vi "Can_File_be_Editted.vi"(0 "Filename":path) -> (1 "File Permissions OK?":bool, 2 "File Status":T1=enum."Directory structure cannot be created", 3 "Comment String":string="Directory structure cannot be created", 4 "Cannot create directory":path)   [LabVIEW 2010]
uses:
  File_Status.ctl
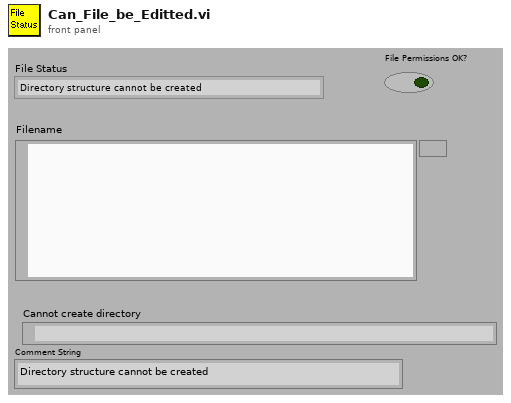
[diagram p1: front panel]
types:
  T1 = typedef "File_Status.ctl" = enum16{"Invalid Path", "This is a folder pathname", "Generic File Error", "Directory structure cannot be created", "File cannot be created", "File can be created", "File exist but read only", "File exist but no access", "File exist with read and write access"}
  T2 = enum16{"read/write", "read-only", "write-only", "write-only (truncate)"}
  T3 = enum16{"open", "replace", "create", "open or create", "replace or create", "replace or create with confirmation"}
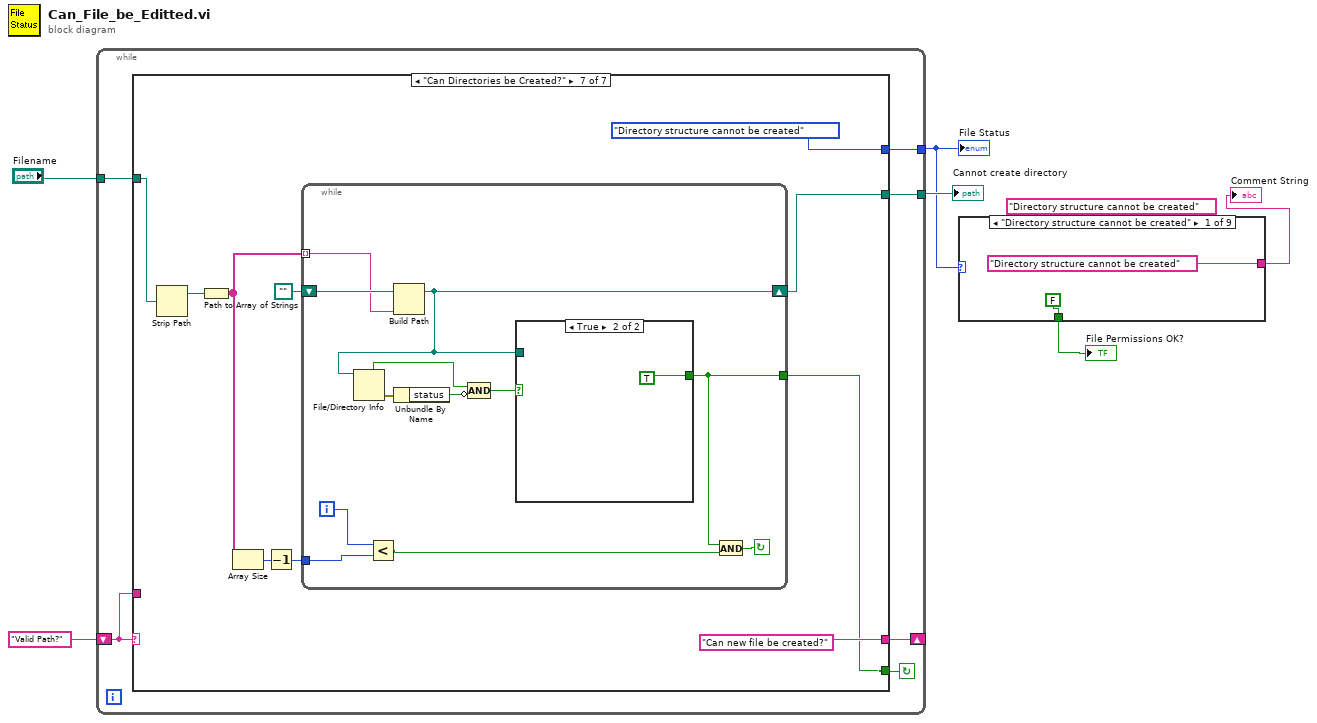
[diagram p0: block diagram]
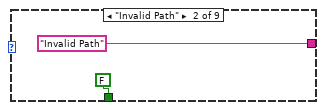
[diagram p2: hidden frame]
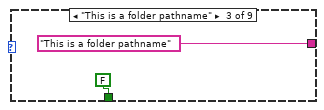
[diagram p3: hidden frame]
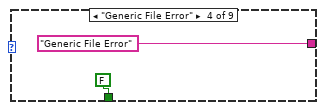
[diagram p4: hidden frame]
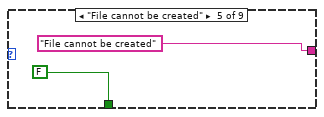
[diagram p5: hidden frame]
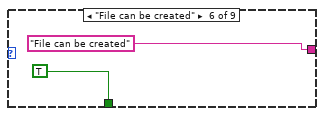
[diagram p6: hidden frame]
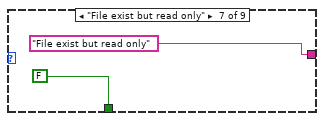
[diagram p7: hidden frame]
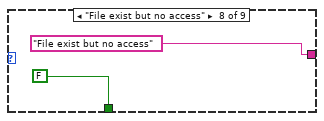
[diagram p8: hidden frame]
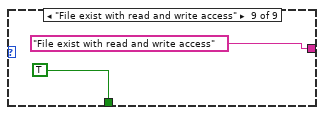
[diagram p9: hidden frame]
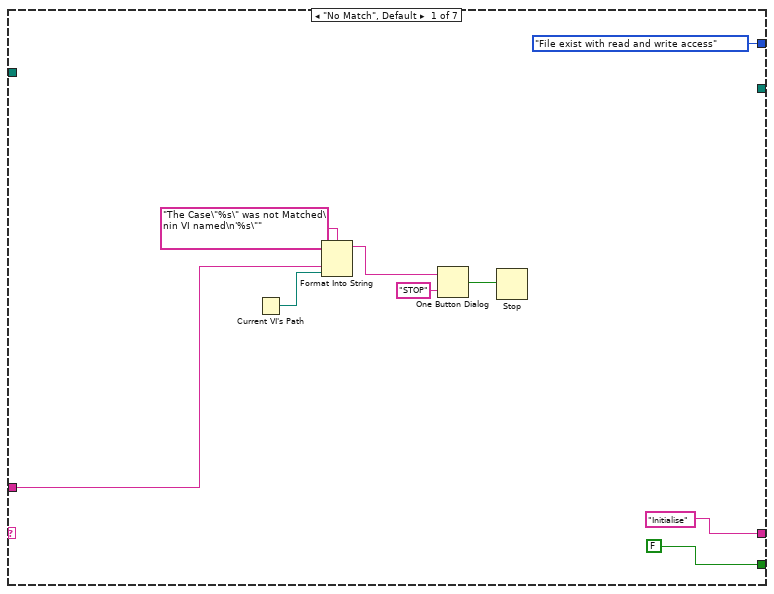
[diagram p10: hidden frame]
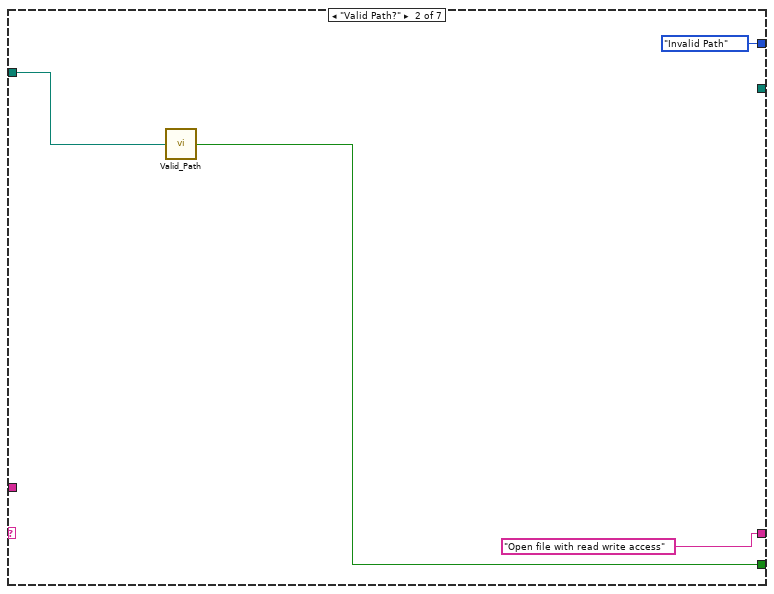
[diagram p11: hidden frame]
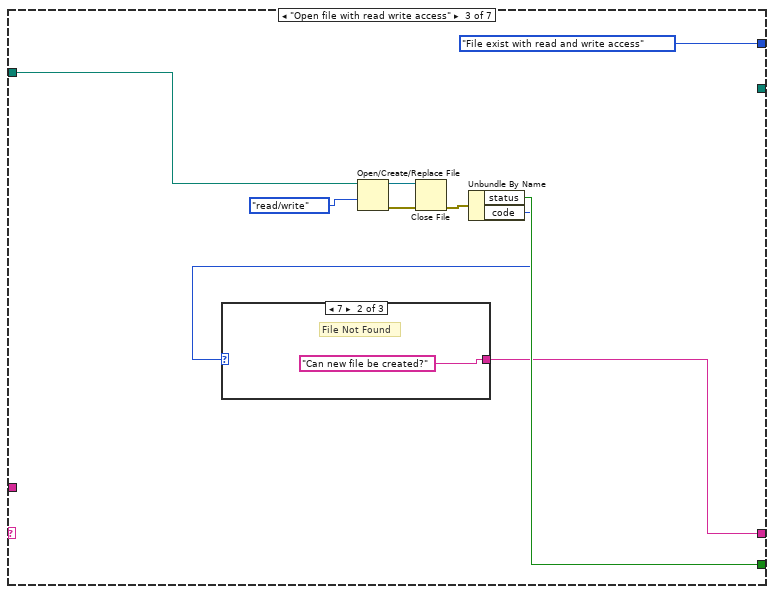
[diagram p12: hidden frame]
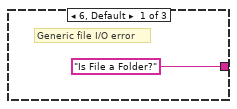
[diagram p13: hidden frame]
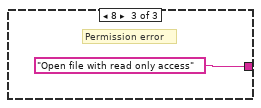
[diagram p14: hidden frame]
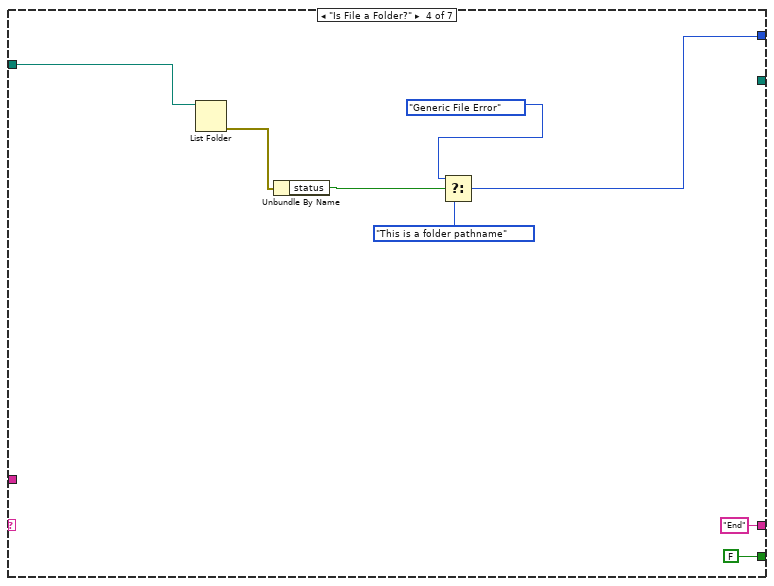
[diagram p15: hidden frame]
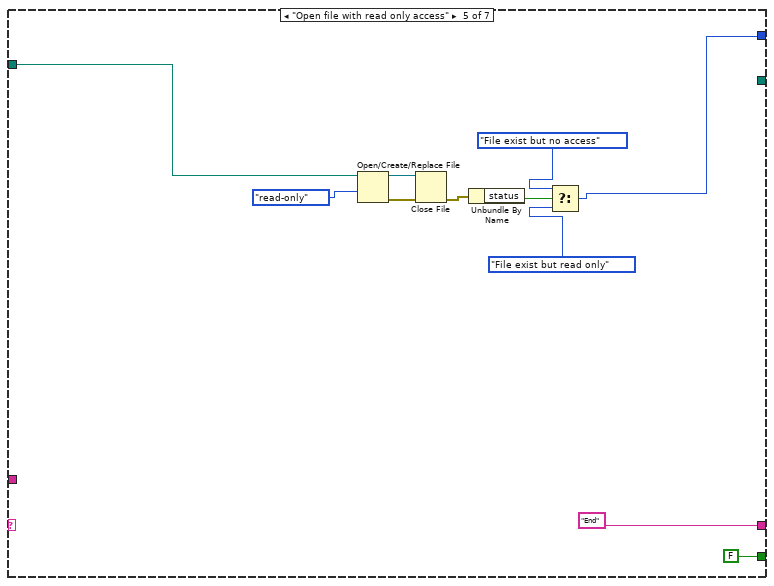
[diagram p16: hidden frame]
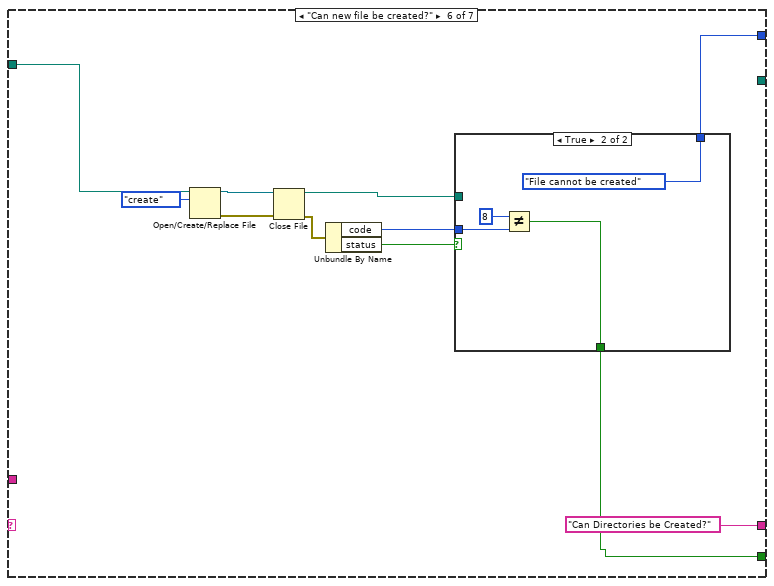
[diagram p17: hidden frame]
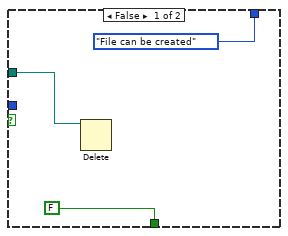
[diagram p18: hidden frame]
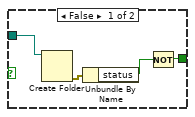
[diagram p19: hidden frame]
diagram:
  (unwired) "Directory structure cannot be created"
  n1 = while {
    shift-left: "Valid Path?" -> [w10]
    shift-right: [w11] -> _
    tunnel: "Filename" -> [w9]
    tunnel: [w8] -> w4
    tunnel: [w7] -> w5
    stop <- w12 continue-if-true
    n2 = case shown="\"Can Directories be Created?\"" w10 {
      tunnel: [FALSE w23 w29 FALSE ("status") FALSE ("status") w60 w76] -> w12
      tunnel: ["Initialise" "Open file with read write access" w26 "End" ("f") "End" "Can Directories be Created?" "Can new file be created?"] -> w11
      tunnel: w10 -> [w16 _ _ _ _ _ _]
      tunnel: w9 -> [_ w24 w31 w45 w51 w62 w82]
      tunnel: [File_Status."File exist with read and write access" ("File Status") File_Status."Invalid Path" ("File Status") File_Status."File exist with read and write access" ("File Status") w38 w46 w58 File_Status."Directory structure cannot be created" ("File Status")] -> w8
      tunnel: [_ _ _ _ _ _ w75] -> w7
      frame "No Match", Default {
        n3 = Current VI's Path() -> (path=w15:path)
        n4 = Format Into String(format string="The Case\"%s\" was not Matched\nin VI named\n'%s\"" ("Format String"), w16, w15) -> (resulting string=w19:string)  [unwired: 2 in, 1 out]
        n5 = One Button Dialog(message=w19, button name ("OK")="STOP") -> (true=w17:bool)
        n6 = Stop(stop? (T)=w17) -> ()
      }
      frame "Valid Path?" {
        n7 = call "Valid_Path.vi"("Filename"=w24) -> ("Valid Path?"=w23:bool)
      }
      frame "Open file with read write access" {
        n8 = Open/Create/Replace File(file path (use dialog)=w31, access (0:read/write)=T2."read/write" ("open mode (0)")) -> (refnum out=w32:refnum<file>, error out=w34:errorcluster)  [unwired: 1 in, 4 out]
        n9 = Close File(refnum=w32, error in=w34) -> (error out=w28:errorcluster)  [unwired: 1 out]
        n10 = Unbundle By Name(w28) -> ("status"=w29:bool, "code"=w27:i32)
        n11 = case shown="7" w27 {
          tunnel: ["Is File a Folder?" ("f") "Can new file be created?" ("f") "Open file with read only access"] -> w26
          frame 6, Default {
            # "Generic file I/O error"
          }
          frame 7 {
            # "File Not Found"
          }
          frame 8 {
            # "Permission error"
          }
        }
      }
      frame "Is File a Folder?" {
        n12 = List Folder(path=w45) -> (error out=w44:errorcluster)  [unwired: 1 in, 5 out]
        n13 = Unbundle By Name(w44) -> ("status"=w41:bool)
        n14 = Select(t=File_Status."Generic File Error" ("File Status"), s=w41, f=File_Status."This is a folder pathname" ("File Status")) -> (s? t:f=w38:T1)
      }
      frame "Open file with read only access" {
        n15 = Open/Create/Replace File(file path (use dialog)=w51, access (0:read/write)=T2."read-only" ("open mode (0)")) -> (refnum out=w52:refnum<file>, error out=w55:errorcluster)  [unwired: 1 in, 4 out]
        n16 = Close File(refnum=w52, error in=w55) -> (error out=w54:errorcluster)  [unwired: 1 out]
        n17 = Unbundle By Name(w54) -> ("status"=w49:bool)
        n18 = Select(t=File_Status."File exist but no access" ("File Status"), s=w49, f=File_Status."File exist but read only" ("File Status")) -> (s? t:f=w46:T1)
      }
      frame "Can new file be created?" {
        n19 = Open/Create/Replace File(file path (use dialog)=w62, operation (0:open)=T3."create") -> (refnum out=w66:refnum<file>, error out=w65:errorcluster)  [unwired: 1 in, 4 out]
        n20 = Close File(refnum=w66, error in=w65) -> (path=w61:path, error out=w64:errorcluster)
        n21 = Unbundle By Name(w64) -> ("code"=w59:i32, "status"=w63:bool)
        n22 = case shown="True" w63 {
          tunnel: w61 -> [w70 _]
          tunnel: [FALSE w71] -> w60
          tunnel: w59 -> [_ w74]
          tunnel: [File_Status."File can be created" ("File Status") File_Status."File cannot be created" ("File Status")] -> w58
          frame False {
            n23 = Delete(path (use dialog)=w70) -> ()  [unwired: 1 in, 6 out]
          }
          frame True {
            n24 = Not Equal?(x=8, y=w74) -> (x != y?=w71:bool)
          }
        }
      }
      frame "Can Directories be Created?" {
        n25 = Strip Path(path=w82) -> (stripped path=w77:path)  [unwired: 1 out]
        n26 = Path to Array of Strings(0:w77) -> (2:w79:string[])  [unwired: 1 out]
        n27 = Array Size(array=w79) -> (size(s)=w81:i32)
        n28 = Decrement(x=w81) -> (x-1=w80:i32)
        n29 = while {
          tunnel: [w91] -> w76
          tunnel: w80 -> [w94]
          shift-left: path "" ("appended path") -> [w96]
          shift-right: [w90] -> w75
          tunnel: w79 -> [w95] mode=indexing
          i -> [w85]
          stop <- w92 continue-if-true
          n30 = Less?(x=w85, y=w94) -> (x < y?=w93:bool)
          n31 = Build Path(base path=w96, name or relative path=w95) -> (appended path=w90:path)
          n32 = File/Directory Info(path=w90) -> (directory=w87:bool, error out=w89:errorcluster)  [unwired: 1 in, 5 out]
          n33 = Unbundle By Name(w89) -> ("status"=w88:bool)
          n34 = Compound Arithmetic op=AND(w87, invert w88) -> (w86:bool)
          n35 = case shown="True" w86 {
            tunnel: w90 -> [w100 _]
            tunnel: [w97 TRUE] -> w91
            frame False {
              n36 = Create Folder(path (use dialog)=w100) -> (error out=w99:errorcluster)  [unwired: 1 in, 3 out]
              n37 = Unbundle By Name(w99) -> ("status"=w98:bool)
              n38 = Not(x=w98) -> (.not. x?=w97:bool)
            }
            frame True {
            }
          }
          n39 = And(x=w91, y=w93) -> (x .and. y?=w92:bool)
        }
      }
    }
  }
  "File Status" <- w4
  "Cannot create directory" <- w5
  n40 = case shown="\"Directory structure cannot be created\"" w4 {
    tunnel: [FALSE FALSE FALSE FALSE FALSE TRUE FALSE FALSE TRUE] -> w3
    tunnel: ["Directory structure cannot be created" "Invalid Path" "This is a folder pathname" "Generic File Error" "File cannot be created" "File can be created" "File exist but read only" "File exist but no access" "File exist with read and write access"] -> w2
    frame "Directory structure cannot be created" {
    }
    frame "Invalid Path" {
    }
    frame "This is a folder pathname" {
    }
    frame "Generic File Error" {
    }
    frame "File cannot be created" {
    }
    frame "File can be created" {
    }
    frame "File exist but read only" {
    }
    frame "File exist but no access" {
    }
    frame "File exist with read and write access" {
    }
  }
  "File Permissions OK?" <- w3
  "Comment String" <- w2
